vi "Apply Audiogram Compensation.vi"(0 "Noise in":refnum<class "Noise.lvclass">, 7 "Noise (flattened!)":dbl[](array[numeric]), 9 "Fs (Hz)":dbl, 11 "error in (no error)":errorcluster) -> (4 "Noise out":refnum<class "Noise.lvclass">, 8 "Compensated":dbl[](array[numeric]), 10 "Gain":dbl, 15 "error out":errorcluster)   [LabVIEW 2020, in "Noise.lvclass"]
uses:
  Noise.lvclass
  Noise.lvclass/Noise.ctl
  d0102e83-39f4-47be-9330-e3a2bf791250.vi
  20976c62-2d82-48eb-9cd9-aa73218fb8d2.vi
  Utility VIs/Math VIs/FFT x(t) to dB,Degrees (1D).vi
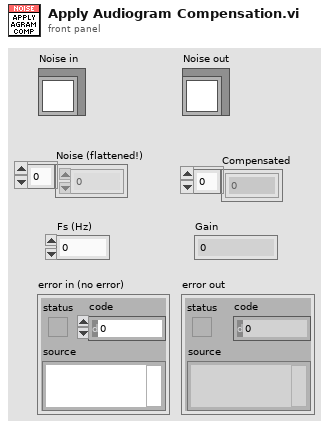
[diagram p1: front panel]
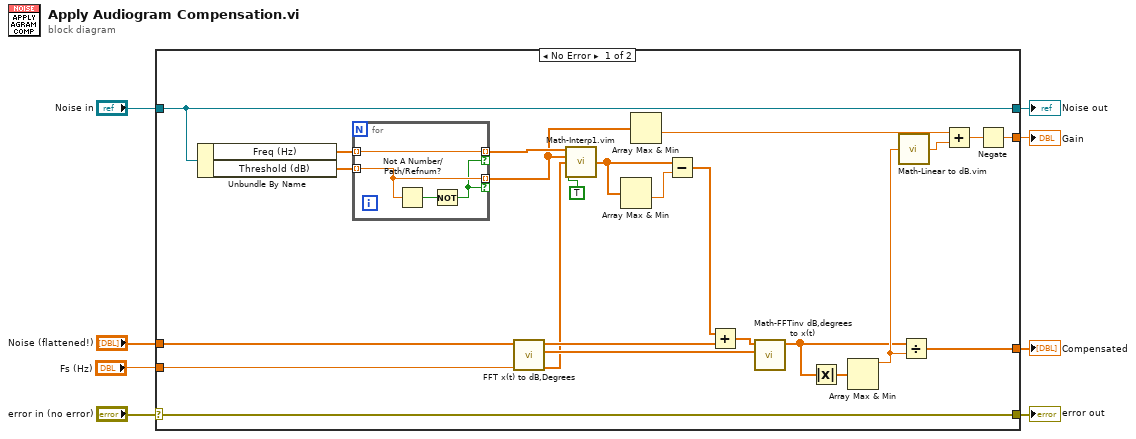
[diagram p0: block diagram]
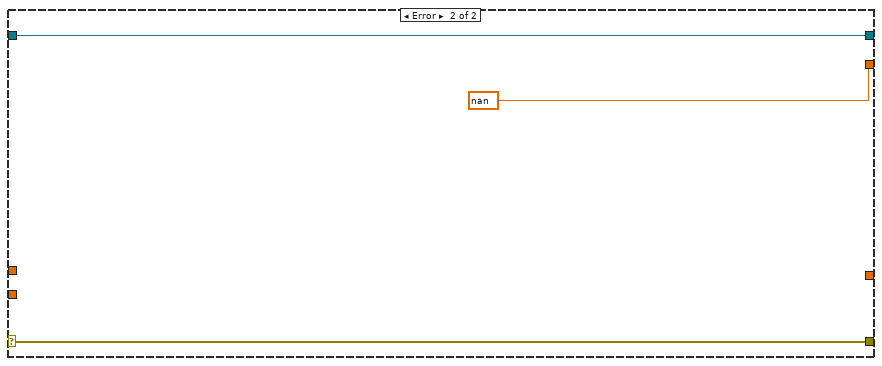
[diagram p2: hidden frame]
diagram:
  n1 = case shown="No Error" "error in (no error)" {
    selector: "error in (no error)" -> [w32 w39]
    tunnel: [w32 w39] -> w7
    tunnel: [w27 w38] -> w5
    tunnel: "Noise in" -> [w27 w38]
    tunnel: "Fs (Hz)" -> [w12 _]
    tunnel: [w9 nan] -> w1
    tunnel: [w29 _] -> w3
    tunnel: "Noise (flattened!)" -> [w26 _]
    frame No Error {
      n2 = Unbundle By Name(w27) -> ("Freq (Hz)"=w25:dbl[], "Threshold (dB)"=w24:dbl[])
      n3 = for {
        tunnel: w25 -> [w36] mode=indexing
        tunnel: w24 -> [w35] mode=indexing
        tunnel: [w36] -> w22 mode=indexing if=w33
        tunnel: [w35] -> w16 mode=indexing if=w33
        n4 = Not A Number/Path/Refnum?(number/path/refnum=w35) -> (NaN/Path/Refnum?=w34:bool)
        n5 = Not(x=w34) -> (.not. x?=w33:bool)
      }
      n6 = call-poly "FFT x(t) to dB,Degrees.vi"("Fs (Hz)"=w12, "X"=w26) -> ("Freq (Hz)"=w11:dbl[], "+Freq Phase of FFT (degrees)"=w23:dbl[], "+Freq. Mag of FFT (dB rms)"=w13:dbl[])  [unwired: 7 in]
      n7 = call "Math-Interp1.vim"("X"=w22, "Y"=w16, "U"=w11, "extrapolate (T)"=TRUE ("extrapolate")) -> ("V"=w20:dbl[])  [unwired: 11 in]
      n8 = Array Max & Min(array=w20) -> (min value=w19:dbl)  [unwired: 3 out]
      n9 = Array Max & Min(array=w16) -> (min value=w15:dbl)  [unwired: 3 out]
      n10 = Subtract(x=w20, y=w19) -> (x-y=w10:dbl[])
      n11 = Add(x=w10, y=w13) -> (x+y=w14:dbl[])
      n12 = call "Math-FFTinv dB,degrees to x(t).vi"("+Freq Phase of FFT (degrees)"=w23, "+Freq. Mag of FFT (rms dB)"=w14) -> ("X(t)"=w28:dbl[])  [unwired: 8 in, 1 out]
      n13 = Absolute Value(x=w28) -> (abs(x)=w31:dbl[])
      n14 = Array Max & Min(array=w31) -> (max value=w30:dbl)  [unwired: 3 out]
      n15 = call "Math-Linear to dB.vim"("linear"=w30) -> ("dB"=w17:dbl)
      n16 = Divide(x=w28, y=w30) -> (x/y=w29:dbl[])
      n17 = Add(x=w15, y=w17) -> (x+y=w18:dbl)
      n18 = Negate(x=w18) -> (-x=w9:dbl)
    }
    frame Error {
    }
  }
  "error out" <- w7
  "Noise out" <- w5
  "Gain" <- w1
  "Compensated" <- w3
